vi "Write ProjectName.vi"(10 "ProjectName":string, 11 "Project in":refnum<class "Project.lvclass">) -> (3 "Project out":refnum<class "Project.lvclass">)   [LabVIEW 2021, in "Bananas.lvlib" / "Project.lvclass"]
uses:
  Project.lvclass
  Project.lvclass/Project.ctl
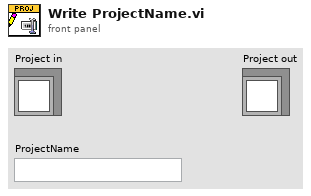
[diagram p1: front panel]
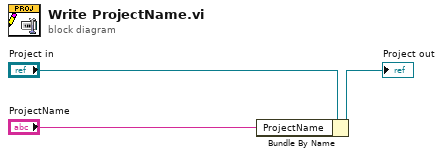
[diagram p0: block diagram]
diagram:
  n1 = Bundle By Name(cluster="Project in", "ProjectName"="ProjectName") -> (→"Project out":refnum<class "Project.lvclass">)
